vi "iTacho_Find Complete Frame-test_harness.vi"(11 "test case ID":string) -> (3 "result":bool)   [LabVIEW 2018]
uses:
  Libraries/iTacho_class/iTacho.lvclass
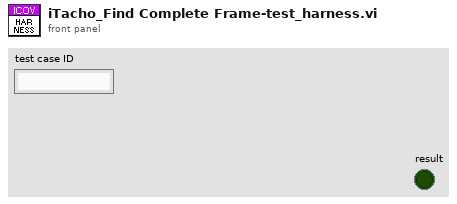
[diagram p1: front panel]
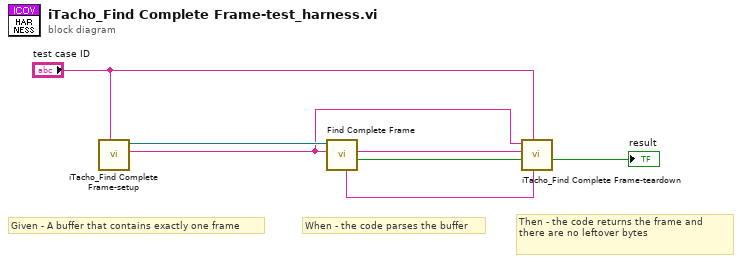
[diagram p0: block diagram]
diagram:
  # "Then - the code returns the frame and there are no leftover bytes"
  # "When - the code parses the buffer"
  # "Given - A buffer that contains exactly one frame"
  n1 = call "iTacho_Find Complete Frame-setup.vi"("test case ID"="test case ID") -> ("Read Buffer"=w4:string, "iTacho"=w5:refnum<class "iTacho.lvclass">)  [unwired: 9 in]
  n2 = call-dynamic "Find Complete Frame.vi"("Read Buffer in"=w4, "iTacho in"=w5) -> ("Found New Frame?"=w2:bool, "Frame"=w3:string, "Leftover Bytes"=w1:string)  [unwired: 5 in, 2 out]
  n3 = call "iTacho_Find Complete Frame-teardown.vi"("Leftover Bytes"=w1, "test case ID"="test case ID", "Found New Frame"=w2, "Actual Frame"=w3, "Expected Frame"=w4) -> ("result"=→"result":bool)  [unwired: 6 in]
